vi "_Remote Park Mass.vi"(4 "UseDefault (F)":bool, 5 "Q2 Park Mass":dbl=400.0 format="%#.3f", 6 "Q1 Park Mass":dbl=400.0 format="%#.3f", 7 "M1RF":dbl=100.0 format="%#.3f") -> (0 "error out":errorcluster, 1 "Q2 Park Mass Out":dbl=400.0 format="%#.3f", 2 "Q1 Park Mass Out":dbl=400.0 format="%#.3f", 3 "M1RF Out":dbl=400.0 format="%#.3f")   [LabVIEW 2015]
uses:
  Type/_RT Active Ch.ctl
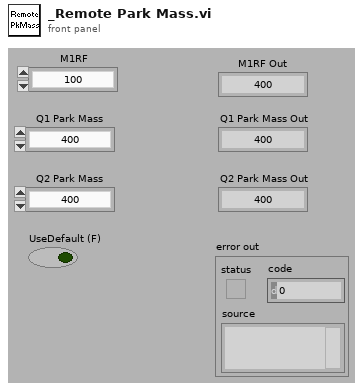
[diagram p1: front panel]
types:
  T1 = typedef "_RT Active Ch.ctl" = cluster{"Start":i32, "Step":i32, "ChID":i32}
  T2 = typedef "_RT Configuration 2.ctl" = cluster{"Name":string, "Ch#":u8, "Min":dbl, "Max":dbl, "Def+":dbl, "Def-":dbl, "Offset":dbl, "Slope":dbl, "Type":u8, "Description":string, "SettleT":dbl}
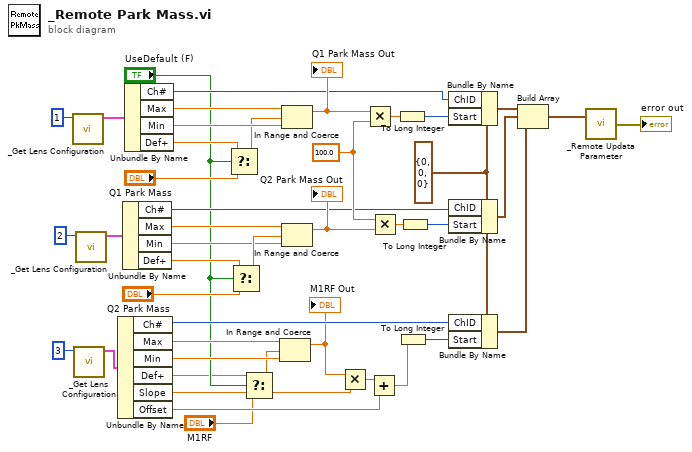
[diagram p0: block diagram]
diagram:
  w10 = T1 {"Start"=0, "Step"=0, "ChID"=0} ("Active Channel")
  w26 = 100.0 ("y")
  n1 = call "_Get Lens Configuration.vi"("Channel #"=u8 1) -> ("Lens Configuration"=w42:T2)  [unwired: 1 in, 5 out]
  n2 = call "_Get Lens Configuration.vi"("Channel #"=u8 3) -> ("Lens Configuration"=w16:T2)  [unwired: 1 in, 5 out]
  n3 = call "_Get Lens Configuration.vi"("Channel #"=u8 2) -> ("Lens Configuration"=w41:T2)  [unwired: 1 in, 5 out]
  n4 = Unbundle By Name(w16) -> ("Ch#"=w12:u8, "Max"=w15:dbl, "Min"=w14:dbl, "Def+"=w3:dbl, "Slope"=w7:dbl, "Offset"=w6:dbl)
  n5 = Unbundle By Name(w41) -> ("Ch#"=w21:u8, "Max"=w33:dbl, "Min"=w31:dbl, "Def+"=w38:dbl)
  n6 = Unbundle By Name(w42) -> ("Ch#"=w23:u8, "Max"=w36:dbl, "Min"=w35:dbl, "Def+"=w40:dbl)
  n7 = Select(t=w40, s="UseDefault (F)", f="Q1 Park Mass") -> (s? t:f=w34:dbl)
  n8 = Select(t=w38, s="UseDefault (F)", f="Q2 Park Mass") -> (s? t:f=w32:dbl)
  n9 = Select(t=w3, s="UseDefault (F)", f="M1RF") -> (s? t:f=w1:dbl)
  n10 = In Range and Coerce(upper limit=w15, x=w1, lower limit=w14) -> (coerced(x)=w8:dbl)  [unwired: 1 out]
  "M1RF Out" <- w8
  n11 = In Range and Coerce(upper limit=w36, x=w34, lower limit=w35) -> (coerced(x)=w28:dbl)  [unwired: 1 out]
  "Q1 Park Mass Out" <- w28
  n12 = In Range and Coerce(upper limit=w33, x=w32, lower limit=w31) -> (coerced(x)=w27:dbl)  [unwired: 1 out]
  "Q2 Park Mass Out" <- w27
  n13 = Multiply(x=w8, y=w7) -> (x*y=w9:dbl)
  n14 = Multiply(x=w28, y=w26) -> (x*y=w29:dbl)
  n15 = Add(x=w9, y=w6) -> (x+y=w5:dbl)
  n16 = Multiply(x=w26, y=w27) -> (x*y=w30:dbl)
  n17 = To Long Integer(number=w29) -> (32bit integer=w24:i32)
  n18 = To Long Integer(number=w5) -> (32bit integer=w13:i32)
  n19 = To Long Integer(number=w30) -> (32bit integer=w22:i32)
  n20 = Bundle By Name(cluster=w10, "ChID"=w23, "Start"=w24) -> (w25:T1)
  n21 = Bundle By Name(cluster=w10, "ChID"=w21, "Start"=w22) -> (w20:T1)
  n22 = Bundle By Name(cluster=w10, "ChID"=w12, "Start"=w13) -> (w11:T1)
  n23 = Build Array(w25, w20, w11) -> (w19:T1[])
  n24 = call "_Remote Updata Parameter.vi"("Parameters"=w19) -> ("error out"=→"error out":errorcluster)  [unwired: 1 in]
